vi "report results.vi"(8 "error in":errorcluster, 10 "result":refnum<class "result.lvclass">, 11 "event reporter in":refnum<class "event reporter.lvclass">) -> (0 "error out":errorcluster, 3 "event reporter out":refnum<class "event reporter.lvclass">)   [LabVIEW 2013, in "event reporter.lvclass"]
uses:
  event reporter.lvclass
  result/result.lvclass
  event reporter.lvclass/event reporter.ctl
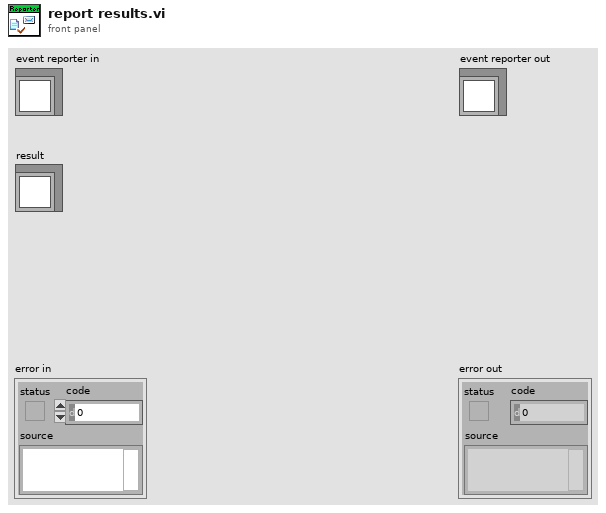
[diagram p1: front panel]
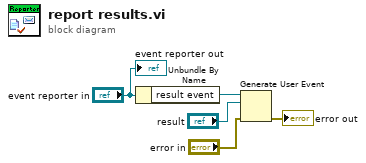
[diagram p0: block diagram]
diagram:
  n1 = Unbundle By Name("event reporter in") -> ("result event"=w1:refnum<user-event>)
  n2 = Generate User Event(user event=w1, event data cluster="result", error in="error in") -> (error out=→"error out":errorcluster)  [unwired: 1 in, 1 out]
  "event reporter out" <- "event reporter in"
